vi "期末專題_R09522534_楊日昌.vi"() -> ()   [LabVIEW 2014]
uses:
  <vilib>/Utility/miscctls.llb/LVPositionTypeDef.ctl
  <vilib>/Utility/inputDevices.llb/keyboardAcquire.vi
panel:
  out "test":dbl
  out "撞擊次數2":dbl
  out "撞擊次數1":dbl
  out "操作模式":string
  out "操作模式":string
  in  "stop":bool
  out "Ball 3":bool
  out "Ball 2":bool
  out "最佳成績":dbl
  out "judge2":dbl
  out "分數":dbl
  out "選擇的模式2":dbl
  out "judge1":dbl
  out "選擇的模式1":dbl
  in  "Boolean":bool=TRUE
  out "bowling5":bool=TRUE
  out "bowling4":bool=TRUE
  out "時間":dbl
  out "Ball":bool=TRUE
  out "碰撞次數(以內)":dbl
  out "bowling3":bool=TRUE
  out "bowling2":bool=TRUE
  in  "START":bool
  out "bowling1":bool=TRUE
  in  "Dial":dbl(knob)
  # "保齡撞撞樂"
  # "加分任務"
  # "操作及模式"
  # "出球"
  # "移動"
  # "角度"
  # "操作模式"
  # ":"
  # "剩餘球數"
types:
  T1 = typedef "LVPositionTypeDef.ctl" = cluster{"Left":i32, "Top":i32}
  T2 = enum16{"0", "1", "2", "3", "4", "5", "6", "7", "8", "9", "A", "B", "C", "D", "E", "F", "G", "H", "I", "J", "K", "L", "M", "N", "O", "P", "Q", "R", "S", "T", "U", "V", "W", "X", "Y", "Z", "F1", "F2", "F3", "F4", "F5", "F6", "F7", "F8", "F9", "F10", "F11", "F12", "F13", "F14", "F15", "ADD", "BACK", "BACKSLASH", "CAPITAL", "COMMA", "DECIMAL", "DELETE", "DIVIDE", "DOWN", "END", "EQUALS", "ESCAPE", "GRAVE (`)", "HOME", "INSERT", "LBRACKET", "LCONTROL", "LEFT", "L ALT", "LSHIFT", "LWIN", "MINUS", "MULTIPLY", "NEXT", "NUMLOCK", "NUMPAD_0", "NUMPAD_1", "NUMPAD_2", "NUMPAD_3", "NUMPAD_4", "NUMPAD_5", "NUMPAD_6", "NUMPAD_7", "NUMPAD_8", "NUMPAD_9", "PAUSE", "PERIOD", "PRIOR (PG UP)", "RBRACKET", "RCONTROL", "RETURN", "RIGHT", "R ALT", "RSHIFT", "RWIN", "SCROLL", "SEMICOLON", "SLASH", "SPACE", "SUBTRACT", "TAB", "UP", "ENTER (num pad)", "' (quote)"}[]
  T3 = enum16{"0", "1", "2", "3", "4", "5", "6", "7", "8", "9", "A", "B", "C", "D", "E", "F", "G", "H", "I", "J", "K", "L", "M", "N", "O", "P", "Q", "R", "S", "T", "U", "V", "W", "X", "Y", "Z", "F1", "F2", "F3", "F4", "F5", "F6", "F7", "F8", "F9", "F10", "F11", "F12", "F13", "F14", "F15", "ADD", "BACK", "BACKSLASH", "CAPITAL", "COMMA", "DECIMAL", "DELETE", "DIVIDE", "DOWN", "END", "EQUALS", "ESCAPE", "GRAVE (`)", "HOME", "INSERT", "LBRACKET", "LCONTROL", "LEFT", "L ALT", "LSHIFT", "LWIN", "MINUS", "MULTIPLY", "NEXT", "NUMLOCK", "NUMPAD_0", "NUMPAD_1", "NUMPAD_2", "NUMPAD_3", "NUMPAD_4", "NUMPAD_5", "NUMPAD_6", "NUMPAD_7", "NUMPAD_8", "NUMPAD_9", "PAUSE", "PERIOD", "PRIOR (PG UP)", "RBRACKET", "RCONTROL", "RETURN", "RIGHT", "R ALT", "RSHIFT", "RWIN", "SCROLL", "SEMICOLON", "SLASH", "SPACE", "SUBTRACT", "TAB", "UP", "ENTER (num pad)", "' (quote)"}
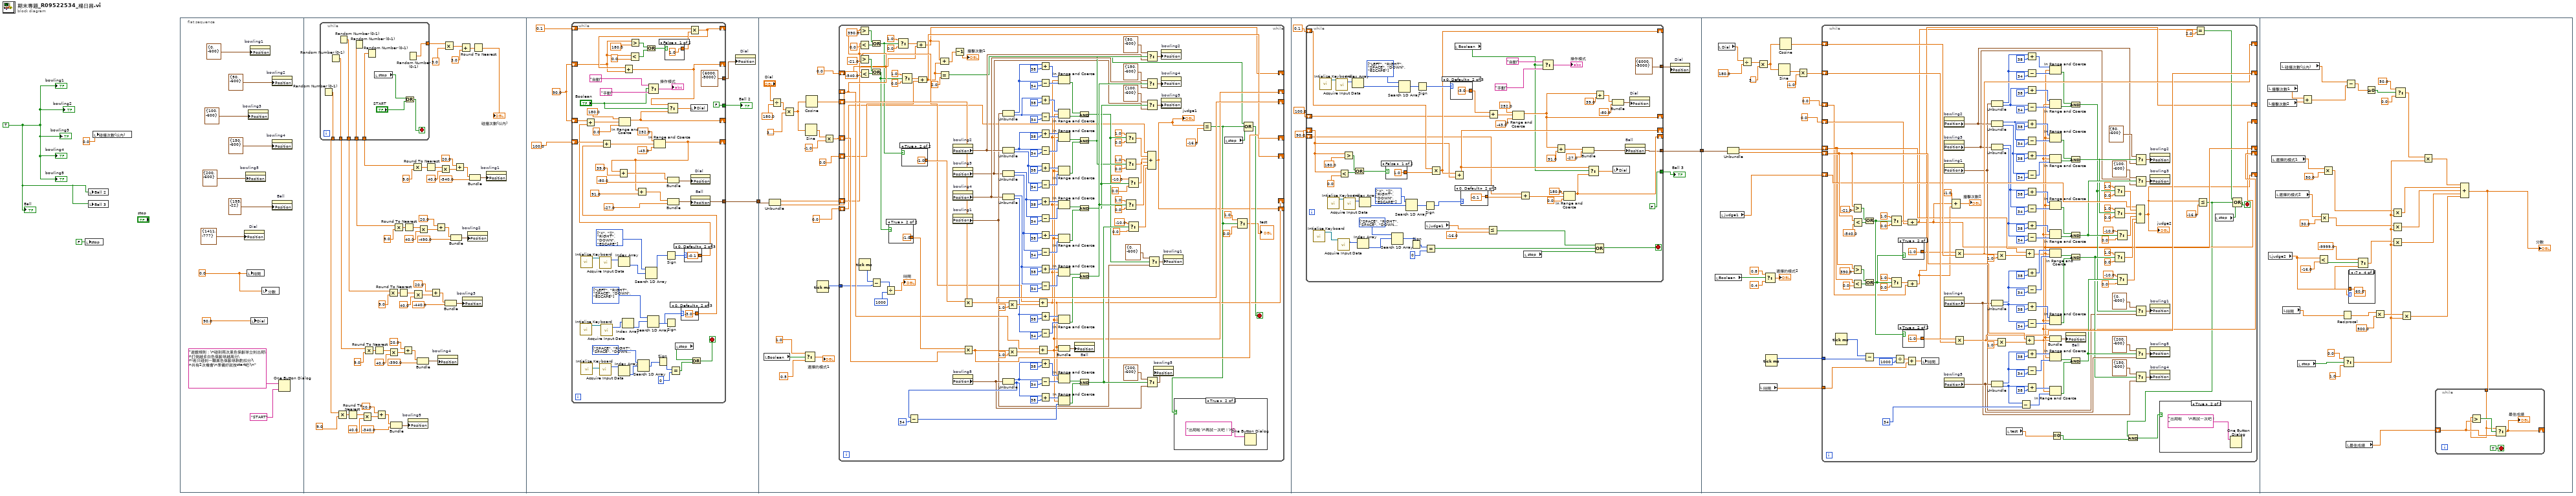
[diagram p0: block diagram]
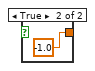
[diagram p2: hidden frame]
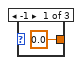
[diagram p3: hidden frame]
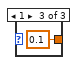
[diagram p4: hidden frame]
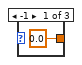
[diagram p5: hidden frame]
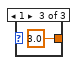
[diagram p6: hidden frame]
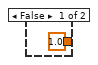
[diagram p8: hidden frame]
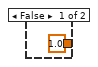
[diagram p9: hidden frame]
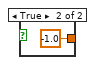
[diagram p10: hidden frame]
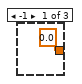
[diagram p11: hidden frame]
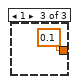
[diagram p12: hidden frame]
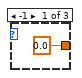
[diagram p13: hidden frame]
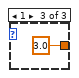
[diagram p14: hidden frame]
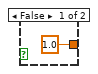
[diagram p16: hidden frame]
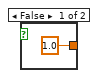
[diagram p17: hidden frame]
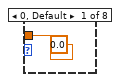
[diagram p18: hidden frame]
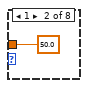
[diagram p19: hidden frame]
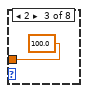
[diagram p20: hidden frame]
diagram:
  w1 = TRUE
  n1 = local write "stop"(FALSE ("stop")) -> ()
  n2 = local write "Ball 2"(w1) -> ()
  n3 = local write "Ball 3"(w1) -> ()
  n4 = local write "碰撞次數(以內)"(0.0 ("Bouncing")) -> ()
  n5 = flat-sequence {
    tunnel: [w86] -> w5
    tunnel: w5 -> [w174]
    tunnel: [w329] -> w4
    tunnel: w4 -> [w414]
    frame #0 {
      w8 = 0.0 ("Time")
      n6 = property on="Dial" class="Knob (strict)"("Position"=T1 {"Left"=1411, "Top"=-777}) -> ()  [unwired: 2 in, 2 out]
      n7 = property on="bowling5" class="Bool (strict)"("Position"=T1 {"Left"=200, "Top"=-600}) -> ()  [unwired: 2 in, 2 out]
      n8 = local write "時間"(w8) -> ()
      n9 = property on="bowling3" class="Bool (strict)"("Position"=T1 {"Left"=100, "Top"=-600}) -> ()  [unwired: 2 in, 2 out]
      n10 = property on="bowling1" class="Bool (strict)"("Position"=T1 {"Left"=0, "Top"=-600}) -> ()  [unwired: 2 in, 2 out]
      n11 = local write "Dial"(90.0 ("Gauge")) -> ()
      n12 = local write "分數"(w8) -> ()
      n13 = property on="bowling2" class="Bool (strict)"("Position"=T1 {"Left"=50, "Top"=-600}) -> ()  [unwired: 2 in, 2 out]
      n14 = property on="bowling4" class="Bool (strict)"("Position"=T1 {"Left"=150, "Top"=-600}) -> ()  [unwired: 2 in, 2 out]
      n15 = property on="Ball" class="Bool (strict)"("Position"=T1 {"Left"=195, "Top"=-22}) -> ()  [unwired: 2 in, 2 out]
      n16 = One Button Dialog(message="遊戲規則：\n碰到兩次黑色保齡球立刻出局\n打倒越多白色保齡球越高分\n(若只碰到一顆黑色保齡球斟酌扣分)\n共有2次機會\n準備好就按start吧!\n" ("String"), button name ("OK")="START") -> ()  [unwired: 1 out]
    }
    frame #1 {
      n17 = while {
        tunnel: [w81] -> w49
        tunnel: [w80] -> w51
        tunnel: [w79] -> w50
        tunnel: [w78] -> w41
        tunnel: [w77] -> w18
        tunnel: [w76] -> w17
        stop <- w73 stop-if-true
        n18 = Random Number (0-1)() -> (number: 0 to 1=w76:dbl)
        n19 = Random Number (0-1)() -> (number: 0 to 1=w77:dbl)
        n20 = Random Number (0-1)() -> (number: 0 to 1=w80:dbl)
        n21 = Random Number (0-1)() -> (number: 0 to 1=w79:dbl)
        n22 = Random Number (0-1)() -> (number: 0 to 1=w81:dbl)
        n23 = local read "stop"() -> (w75:bool)
        n24 = Or(x=w75, y="START") -> (x .or. y?=w73:bool)
        n25 = Random Number (0-1)() -> (number: 0 to 1=w78:dbl)
      }
      n26 = Multiply(x=w17, y=9.0) -> (x*y=w22:dbl)
      n27 = Round To Nearest(number=w22) -> (nearest integer value=w21:dbl)
      n28 = Multiply(x=w21, y=40.0) -> (x*y=w25:dbl)
      n29 = Multiply(x=w18, y=9.0) -> (x*y=w35:dbl)
      n30 = Round To Nearest(number=w35) -> (nearest integer value=w36:dbl)
      n31 = Add(x=20.0, y=w25) -> (x+y=w26:dbl)
      n32 = Multiply(x=w51, y=9.0) -> (x*y=w44:dbl)
      n33 = Multiply(x=w36, y=40.0) -> (x*y=w32:dbl)
      n34 = Bundle(w26, "x"=-340.0) -> (w19:cluster{dbl, "x":dbl})  [unwired: 1 in]
      n35 = Multiply(x=w50, y=9.0) -> (x*y=w46:dbl)
      n36 = Round To Nearest(number=w44) -> (nearest integer value=w43:dbl)
      n37 = Add(x=20.0, y=w32) -> (x+y=w31:dbl)
      n38 = Round To Nearest(number=w46) -> (nearest integer value=w45:dbl)
      n39 = property on="bowling5" class="Bool (strict)"("Position"=w19) -> ()  [unwired: 2 in, 2 out]
      n40 = Multiply(x=w49, y=9.0) -> (x*y=w48:dbl)
      n41 = Multiply(x=w43, y=40.0) -> (x*y=w58:dbl)
      n42 = Bundle(w31, "x"=-390.0) -> (w20:cluster{dbl, "x":dbl})  [unwired: 1 in]
      n43 = Multiply(x=w45, y=40.0) -> (x*y=w65:dbl)
      n44 = Round To Nearest(number=w48) -> (nearest integer value=w47:dbl)
      n45 = Add(x=20.0, y=w58) -> (x+y=w59:dbl)
      n46 = Add(x=20.0, y=w65) -> (x+y=w64:dbl)
      n47 = property on="bowling4" class="Bool (strict)"("Position"=w20) -> ()  [unwired: 2 in, 2 out]
      n48 = Multiply(x=w47, y=40.0) -> (x*y=w68:dbl)
      n49 = Multiply(x=w41, y=3.0) -> (x*y=w38:dbl)
      n50 = Bundle(w59, "x"=-440.0) -> (w55:cluster{dbl, "x":dbl})  [unwired: 1 in]
      n51 = Bundle(w64, "x"=-490.0) -> (w56:cluster{dbl, "x":dbl})  [unwired: 1 in]
      n52 = Add(x=20.0, y=w68) -> (x+y=w70:dbl)
      n53 = Add(x=w38, y=3.0) -> (x+y=w39:dbl)
      n54 = property on="bowling3" class="Bool (strict)"("Position"=w55) -> ()  [unwired: 2 in, 2 out]
      n55 = property on="bowling2" class="Bool (strict)"("Position"=w56) -> ()  [unwired: 2 in, 2 out]
      n56 = Bundle(w70, "x"=-540.0) -> (w69:cluster{dbl, "x":dbl})  [unwired: 1 in]
      n57 = Round To Nearest(number=w39) -> (nearest integer value=→"碰撞次數(以內)":dbl)
      n58 = property on="bowling1" class="Bool (strict)"("Position"=w69) -> ()  [unwired: 2 in, 2 out]
    }
    frame #2 {
      w83 = 90.0
      n59 = while {
        shift-right: [w93] -> _
        shift-left: 100.0 -> [w104]
        tunnel: [w116] -> w86
        shift-right: [w114] -> _
        shift-left: w83 -> [w103]
        tunnel: [T1 {"Left"=6000, "Top"=-5000} ("Position")] -> w82
        shift-right: [w89] -> _
        shift-left: w83 -> [w100]
        shift-right: [w101] -> _
        shift-left: 0.1 -> [w107]
        tunnel: [FALSE ("Ball 2")] -> w84
        stop <- w95 stop-if-true
        w121 = T2 [enum."SPACE", enum."RIGHT", enum."SPACE", enum."DOWN", enum."ESCAPE"] items=["0", "1", "2", "3", "4", "5", "6", "7", "8", "9", "A", "B", "C", "D", "E", "F", "G", "H", "I", "J", "K", "L", "M", "N", "O", "P", "Q", "R", "S", "T", "U", "V", "W", "X", "Y", "Z", "F1", "F2", "F3", "F4", "F5", "F6", "F7", "F8", "F9", "F10", "F11", "F12", "F13", "F14", "F15", "ADD", "BACK", "BACKSLASH", "CAPITAL", "COMMA", "DECIMAL", "DELETE", "DIVIDE", "DOWN", "END", "EQUALS", "ESCAPE", "GRAVE (`)", "HOME", "INSERT", "LBRACKET", "LCONTROL", "LEFT", "L ALT", "LSHIFT", "LWIN", "MINUS", "MULTIPLY", "NEXT", "NUMLOCK", "NUMPAD_0", "NUMPAD_1", "NUMPAD_2", "NUMPAD_3", "NUMPAD_4", "NUMPAD_5", "NUMPAD_6", "NUMPAD_7", "NUMPAD_8", "NUMPAD_9", "PAUSE", "PERIOD", "PRIOR (PG UP)", "RBRACKET", "RCONTROL", "RETURN", "RIGHT", "R ALT", "RSHIFT", "RWIN", "SCROLL", "SEMICOLON", "SLASH", "SPACE", "SUBTRACT", "TAB", "UP", "ENTER (num pad)", "' (quote)"] ("keys pressed 2")
        w132 = T2 [enum."X", enum."Z", enum."RIGHT", enum."DOWN", enum."ESCAPE"] items=["0", "1", "2", "3", "4", "5", "6", "7", "8", "9", "A", "B", "C", "D", "E", "F", "G", "H", "I", "J", "K", "L", "M", "N", "O", "P", "Q", "R", "S", "T", "U", "V", "W", "X", "Y", "Z", "F1", "F2", "F3", "F4", "F5", "F6", "F7", "F8", "F9", "F10", "F11", "F12", "F13", "F14", "F15", "ADD", "BACK", "BACKSLASH", "CAPITAL", "COMMA", "DECIMAL", "DELETE", "DIVIDE", "DOWN", "END", "EQUALS", "ESCAPE", "GRAVE (`)", "HOME", "INSERT", "LBRACKET", "LCONTROL", "LEFT", "L ALT", "LSHIFT", "LWIN", "MINUS", "MULTIPLY", "NEXT", "NUMLOCK", "NUMPAD_0", "NUMPAD_1", "NUMPAD_2", "NUMPAD_3", "NUMPAD_4", "NUMPAD_5", "NUMPAD_6", "NUMPAD_7", "NUMPAD_8", "NUMPAD_9", "PAUSE", "PERIOD", "PRIOR (PG UP)", "RBRACKET", "RCONTROL", "RETURN", "RIGHT", "R ALT", "RSHIFT", "RWIN", "SCROLL", "SEMICOLON", "SLASH", "SPACE", "SUBTRACT", "TAB", "UP", "ENTER (num pad)", "' (quote)"] ("keys pressed 2")
        w143 = T2 [enum."LEFT", enum."RIGHT", enum."SPACE", enum."DOWN", enum."ESCAPE"] items=["0", "1", "2", "3", "4", "5", "6", "7", "8", "9", "A", "B", "C", "D", "E", "F", "G", "H", "I", "J", "K", "L", "M", "N", "O", "P", "Q", "R", "S", "T", "U", "V", "W", "X", "Y", "Z", "F1", "F2", "F3", "F4", "F5", "F6", "F7", "F8", "F9", "F10", "F11", "F12", "F13", "F14", "F15", "ADD", "BACK", "BACKSLASH", "CAPITAL", "COMMA", "DECIMAL", "DELETE", "DIVIDE", "DOWN", "END", "EQUALS", "ESCAPE", "GRAVE (`)", "HOME", "INSERT", "LBRACKET", "LCONTROL", "LEFT", "L ALT", "LSHIFT", "LWIN", "MINUS", "MULTIPLY", "NEXT", "NUMLOCK", "NUMPAD_0", "NUMPAD_1", "NUMPAD_2", "NUMPAD_3", "NUMPAD_4", "NUMPAD_5", "NUMPAD_6", "NUMPAD_7", "NUMPAD_8", "NUMPAD_9", "PAUSE", "PERIOD", "PRIOR (PG UP)", "RBRACKET", "RCONTROL", "RETURN", "RIGHT", "R ALT", "RSHIFT", "RWIN", "SCROLL", "SEMICOLON", "SLASH", "SPACE", "SUBTRACT", "TAB", "UP", "ENTER (num pad)", "' (quote)"] ("keys pressed 2")
        n60 = call <vilib>:"Intialize Keyboard.vi"() -> ("device ID"=w144:refnum<k1>)  [unwired: 10 in, 1 out]
        n61 = call <vilib>:"Intialize Keyboard.vi"() -> ("device ID"=w125:refnum<k1>)  [unwired: 10 in, 1 out]
        n62 = call <vilib>:"Intialize Keyboard.vi"() -> ("device ID"=w120:refnum<k1>)  [unwired: 10 in, 1 out]
        n63 = call-poly <vilib>:"Acquire Input Data.vi"("device ID"=w120) -> ("keys pressed"=w122:T2)  [unwired: 16 in, 2 out]
        n64 = call-poly <vilib>:"Acquire Input Data.vi"("device ID"=w125) -> ("keys pressed"=w126:T2)  [unwired: 16 in, 2 out]
        n65 = call-poly <vilib>:"Acquire Input Data.vi"("device ID"=w144) -> ("keys pressed"=w142:T2)  [unwired: 16 in, 2 out]
        n66 = Index Array(array=w122) -> (element=w123:T3)  [unwired: 1 in]
        n67 = Index Array(array=w126) -> (element=w124:T3)  [unwired: 1 in]
        n68 = Index Array(array=w142) -> (element=w133:T3)  [unwired: 1 in]
        n69 = Less?(x=w100, y=0.0) -> (x < y?=w111:bool)
        n70 = Greater?(x=w100, y=180.0) -> (0:w110:bool)
        n71 = Search 1D Array(1D array=w121, element=w123) -> (index of element=w119:i32)  [unwired: 1 in]
        n72 = Search 1D Array(1D array=w132, element=w124) -> (index of element=w131:i32)  [unwired: 1 in]
        n73 = Or(x=w110, y=w111) -> (x .or. y?=w108:bool)
        n74 = Search 1D Array(1D array=w143, element=w133) -> (index of element=w145:i32)  [unwired: 1 in]
        n75 = Select(t="自動", s="Boolean", f="手動") -> (s? t:f=→"操作模式":string)
        n76 = Sign(1:w119) -> (0:w118:i32)
        n77 = case shown="False" w108 {
          tunnel: [1.0 -1.0] -> w113
          frame False {
          }
          frame True {
          }
        }
        n78 = Sign(1:w131) -> (0:w127:i32)
        n79 = Sign(1:w145) -> (0:w146:i32)
        n80 = Equal?(x=w118, y=0) -> (x = y?=w96:bool)
        n81 = local read "stop"() -> (w97:bool)
        n82 = case shown="0, Default" w146 {
          tunnel: [0.0 -3.0 3.0] -> w94
          frame -1 {
          }
          frame 0, Default {
          }
          frame 1 {
          }
        }
        n83 = Add(x=w104, y=w94) -> (x+y=w138:dbl)
        n84 = In Range and Coerce(upper limit=252.0, x=w138, lower limit=-43.0) -> (coerced(x)=w93:dbl)  [unwired: 1 out]
        n85 = Add(x=w93, y=39.0) -> (x+y=w105:dbl)
        n86 = Add(x=w93, y=91.0) -> (x+y=w136:dbl)
        n87 = Bundle(w105, -80.0) -> (w137:cluster{dbl, dbl})  [unwired: 1 in]
        n88 = Bundle(w136, -27.0) -> (w116:cluster{dbl, dbl})  [unwired: 1 in]
        n89 = case shown="0, Default" w127 {
          tunnel: [0.0 -0.1 0.1] -> w102
          frame -1 {
          }
          frame 0, Default {
          }
          frame 1 {
          }
        }
        n90 = Add(x=w103, y=w102) -> (x+y=w130:dbl)
        n91 = In Range and Coerce(upper limit=180.0, x=w130, lower limit=0.0) -> (coerced(x)=w114:dbl)  [unwired: 1 out]
        n92 = Multiply(x=w107, y=w113) -> (x*y=w101:dbl)
        n93 = Add(x=w101, y=w100) -> (x+y=w89:dbl)
        n94 = Select(t=w89, s="Boolean", f=w114) -> (s? t:f=w99:dbl)
        n95 = local write "Dial"(w99) -> ()
        n96 = property on="Dial" class="Knob (strict)"("Position"=w137) -> ()  [unwired: 2 in, 2 out]
        n97 = property on="Ball" class="Bool (strict)"("Position"=w116) -> ()  [unwired: 2 in, 2 out]
        n98 = Or(x=w97, y=w96) -> (x .or. y?=w95:bool)
      }
      "Ball 2" <- w84
      n99 = property on="Dial" class="Knob (strict)"("Position"=w82) -> ()  [unwired: 2 in, 2 out]
    }
    frame #3 {
      n100 = local read "Boolean"() -> (w158:bool)
      n101 = Unbundle(w174) -> (w159:dbl, w173:dbl)
      n102 = Divide(x="Dial", y=180.0) -> (x/y=w170:dbl)
      n103 = Multiply(x=w170, y=3.141592653589793) -> (x*y=w168:dbl)
      n104 = Select(t=1.0, s=w158, f=0.5) -> (s? t:f=→"選擇的模式1":dbl)
      n105 = Sine(x=w168) -> (sin(x)=w166:dbl)
      n106 = Cosine(x=w168) -> (cos(x)=w160:dbl)
      n107 = Tick Count (ms)() -> (millisecond timer value=w163:u32)
      n108 = Multiply(x=w166, y=-1.0) -> (x*y=w165:dbl)
      n109 = while {
        shift-right: [w198] -> _
        shift-left: w159 -> [w194]
        shift-right: [w305] -> _
        shift-left: w160 -> [w319]
        shift-right: [w199] -> _
        shift-left: w173 -> [w311]
        shift-right: [w307] -> _
        shift-left: w165 -> [w312]
        shift-right: [w184] -> _
        shift-left: 0.0 ("y") -> [w185]
        tunnel: w163 -> [w287]
        shift-right: [w182] -> _
        shift-left: 0.0 ("f") -> [w192]
        shift-right: [w181] -> _
        shift-left: 0.0 ("f") -> [w190]
        stop <- w186 stop-if-true
        n110 = Greater?(x=w194, y=390.0) -> (0:w321:bool)
        n111 = Less?(x=w194, y=0.0) -> (x < y?=w320:bool)
        n112 = Greater?(x=w311, y=-21.0) -> (0:w315:bool)
        n113 = Tick Count (ms)() -> (millisecond timer value=w288:u32)
        n114 = Less?(x=w311, y=-540.0) -> (x < y?=w314:bool)
        n115 = Or(x=w321, y=w320) -> (x .or. y?=w196:bool)
        n116 = Or(x=w315, y=w314) -> (x .or. y?=w259:bool)
        n117 = Subtract(x=w288, y=w287) -> (x-y=w286:u32)
        n118 = Divide(x=w286, y=u32 1000) -> (x/y=→"時間":dbl)
        n119 = case shown="True" w259 {
          tunnel: [1.0 -1.0] -> w313
          frame False {
          }
          frame True {
          }
        }
        n120 = Select(t=1.0, s=w196, f=0.0) -> (s? t:f=w191:dbl)
        n121 = Select(t=1.0, s=w259, f=0.0) -> (s? t:f=w193:dbl)
        n122 = case shown="True" w196 {
          tunnel: [1.0 -1.0] -> w195
          frame False {
          }
          frame True {
          }
        }
        n123 = Compound Arithmetic op=ADD(w191, w190) -> (w181:dbl)
        n124 = Compound Arithmetic op=ADD(w193, w192) -> (w182:dbl)
        n125 = Equal?(x=w182, y=2.0) -> (x = y?=w187:bool)
        n126 = Compound Arithmetic op=ADD(w181, w182) -> (w180:dbl)
        n127 = property on="bowling2" class="Bool (strict)"() -> ("Position"=w214:T1)  [unwired: 2 in, 2 out]
        n128 = property on="bowling3" class="Bool (strict)"() -> ("Position"=w197:T1)  [unwired: 2 in, 2 out]
        n129 = property on="bowling4" class="Bool (strict)"() -> ("Position"=w241:T1)  [unwired: 2 in, 2 out]
        n130 = property on="bowling1" class="Bool (strict)"() -> ("Position"=w200:T1)  [unwired: 2 in, 2 out]
        n131 = property on="bowling5" class="Bool (strict)"() -> ("Position"=w269:T1)  [unwired: 2 in, 2 out]
        n132 = Decrement(x=w180) -> (x-1=→"撞擊次數1":dbl)
        n133 = Multiply(x=w195, y=w319) -> (x*y=w305:dbl)
        n134 = Multiply(x=w313, y=w312) -> (x*y=w307:dbl)
        n135 = Unbundle(w200) -> ("Left"=w207:i32, "Top"=w212:i32)
        n136 = Unbundle(w214) -> ("Left"=w221:i32, "Top"=w226:i32)
        n137 = Unbundle(w197) -> ("Left"=w234:i32, "Top"=w239:i32)
        n138 = Unbundle(w241) -> ("Left"=w243:i32, "Top"=w242:i32)
        n139 = Unbundle(w269) -> ("Left"=w276:i32, "Top"=w281:i32)
        n140 = Subtract(x=w281, y=34) -> (x-y=w277:i32)
        n141 = Multiply(x=w305, y=1.0) -> (x*y=w306:dbl)
        n142 = Multiply(x=w307, y=1.0) -> (x*y=w308:dbl)
        n143 = Add(x=w194, y=w306) -> (x+y=w198:dbl)
        n144 = Add(x=w311, y=w308) -> (x+y=w199:dbl)
        n145 = Add(x=w207, y=38) -> (x+y=w211:i32)
        n146 = Subtract(x=w207, y=34) -> (x-y=w206:i32)
        n147 = Add(x=w212, y=38) -> (x+y=w210:i32)
        n148 = Subtract(x=w212, y=34) -> (x-y=w208:i32)
        n149 = Add(x=w221, y=38) -> (x+y=w225:i32)
        n150 = Subtract(x=w221, y=34) -> (x-y=w220:i32)
        n151 = Add(x=w226, y=38) -> (x+y=w224:i32)
        n152 = Subtract(x=w226, y=34) -> (x-y=w222:i32)
        n153 = Add(x=w234, y=38) -> (x+y=w238:i32)
        n154 = Subtract(x=w234, y=34) -> (x-y=w233:i32)
        n155 = Add(x=w239, y=38) -> (x+y=w237:i32)
        n156 = Subtract(x=w239, y=34) -> (x-y=w235:i32)
        n157 = Add(x=w243, y=38) -> (x+y=w253:i32)
        n158 = Subtract(x=w243, y=34) -> (x-y=w249:i32)
        n159 = Add(x=w242, y=38) -> (x+y=w252:i32)
        n160 = Subtract(x=w242, y=34) -> (x-y=w250:i32)
        n161 = Add(x=w276, y=38) -> (x+y=w280:i32)
        n162 = Subtract(x=w276, y=34) -> (x-y=w275:i32)
        n163 = Add(x=w281, y=38) -> (x+y=w279:i32)
        n164 = In Range and Coerce(upper limit=w211, x=w198, lower limit=w206) -> (In Range?=w202:bool)  [unwired: 1 out]
        n165 = In Range and Coerce(upper limit=w210, x=w199, lower limit=w208) -> (In Range?=w203:bool)  [unwired: 1 out]
        n166 = In Range and Coerce(upper limit=w225, x=w198, lower limit=w220) -> (In Range?=w216:bool)  [unwired: 1 out]
        n167 = In Range and Coerce(upper limit=w224, x=w199, lower limit=w222) -> (In Range?=w217:bool)  [unwired: 1 out]
        n168 = In Range and Coerce(upper limit=w238, x=w198, lower limit=w233) -> (In Range?=w229:bool)  [unwired: 1 out]
        n169 = In Range and Coerce(upper limit=w237, x=w199, lower limit=w235) -> (In Range?=w230:bool)  [unwired: 1 out]
        n170 = In Range and Coerce(upper limit=w253, x=w198, lower limit=w249) -> (In Range?=w245:bool)  [unwired: 1 out]
        n171 = In Range and Coerce(upper limit=w252, x=w199, lower limit=w250) -> (In Range?=w246:bool)  [unwired: 1 out]
        n172 = Bundle(w198, w199) -> (w304:cluster{dbl, dbl})  [unwired: 1 in]
        n173 = In Range and Coerce(upper limit=w280, x=w198, lower limit=w275) -> (In Range?=w271:bool)  [unwired: 1 out]
        n174 = In Range and Coerce(upper limit=w279, x=w199, lower limit=w277) -> (In Range?=w272:bool)  [unwired: 1 out]
        n175 = property on="Ball" class="Bool (strict)"("Position"=w304) -> ()  [unwired: 2 in, 2 out]
        n176 = And(x=w202, y=w203) -> (x .and. y?=w201:bool)
        n177 = And(x=w216, y=w217) -> (x .and. y?=w215:bool)
        n178 = And(x=w229, y=w230) -> (x .and. y?=w228:bool)
        n179 = And(x=w245, y=w246) -> (x .and. y?=w244:bool)
        n180 = And(x=w271, y=w272) -> (x .and. y?=w264:bool)
        n181 = Select(t=1.0, s=w201, f=0.0) -> (s? t:f=w291:dbl)
        n182 = Select(t=1.0, s=w215, f=0.0) -> (s? t:f=w290:dbl)
        n183 = Select(t=1.0, s=w244, f=0.0) -> (s? t:f=w263:dbl)
        n184 = Select(t=-10.0, s=w228, f=0.0) -> (s? t:f=w289:dbl)
        n185 = Select(t=-10.0, s=w264, f=0.0) -> (s? t:f=w262:dbl)
        n186 = Select(t=T1 {"Left"=50, "Top"=-600}, s=w215, f=w214) -> (s? t:f=w299:T1)
        n187 = Select(t=T1 {"Left"=150, "Top"=-600}, s=w244, f=w241) -> (s? t:f=w261:T1)
        n188 = Select(t=T1 {"Left"=100, "Top"=-600}, s=w228, f=w197) -> (s? t:f=w298:T1)
        n189 = Select(t=T1 {"Left"=200, "Top"=-600}, s=w264, f=w269) -> (s? t:f=w260:T1)
        n190 = Compound Arithmetic op=ADD(w185, w291, w290, w289, w263, w262) -> (w184:dbl)
        "judge1" <- w184
        n191 = Select(t=T1 {"Left"=0, "Top"=-600}, s=w201, f=w200) -> (s? t:f=w302:T1)
        n192 = property on="bowling5" class="Bool (strict)"("Position"=w260) -> ()  [unwired: 2 in, 2 out]
        n193 = property on="bowling2" class="Bool (strict)"("Position"=w299) -> ()  [unwired: 2 in, 2 out]
        n194 = property on="bowling4" class="Bool (strict)"("Position"=w261) -> ()  [unwired: 2 in, 2 out]
        n195 = property on="bowling3" class="Bool (strict)"("Position"=w298) -> ()  [unwired: 2 in, 2 out]
        n196 = property on="bowling1" class="Bool (strict)"("Position"=w302) -> ()  [unwired: 2 in, 2 out]
        n197 = Less Or Equal?(x=w184, y=-16.0) -> (x <= y?=w177:bool)
        n198 = case shown="True" w177 {
          frame False {
          }
          frame True {
            n199 = One Button Dialog(message="出局啦 \n再試一次吧！\n") -> ()  [unwired: 1 in, 1 out]
          }
        }
        n200 = local read "stop"() -> (w188:bool)
        n201 = Select(t=1.0, s=w177, f=0.0) -> (s? t:f=→"test":dbl)
        n202 = Compound Arithmetic op=OR(w187, w177, w188) -> (w186:bool)
      }
    }
    frame #4 {
      w331 = 90.0
      n203 = while {
        shift-right: [w352] -> _
        shift-left: 100.0 -> [w337]
        tunnel: [w335] -> w329
        shift-right: [w363] -> _
        shift-left: w331 -> [w338]
        tunnel: [T1 {"Left"=6000, "Top"=-5000} ("Position")] -> w332
        shift-right: [w364] -> _
        shift-left: w331 -> [w349]
        shift-right: [w350] -> _
        shift-left: 0.1 -> [w356]
        tunnel: [FALSE ("Ball 3")] -> w328
        stop <- w345 stop-if-true
        w370 = T2 [enum."SPACE", enum."RIGHT", enum."SPACE", enum."DOWN", enum."ESCAPE"] items=["0", "1", "2", "3", "4", "5", "6", "7", "8", "9", "A", "B", "C", "D", "E", "F", "G", "H", "I", "J", "K", "L", "M", "N", "O", "P", "Q", "R", "S", "T", "U", "V", "W", "X", "Y", "Z", "F1", "F2", "F3", "F4", "F5", "F6", "F7", "F8", "F9", "F10", "F11", "F12", "F13", "F14", "F15", "ADD", "BACK", "BACKSLASH", "CAPITAL", "COMMA", "DECIMAL", "DELETE", "DIVIDE", "DOWN", "END", "EQUALS", "ESCAPE", "GRAVE (`)", "HOME", "INSERT", "LBRACKET", "LCONTROL", "LEFT", "L ALT", "LSHIFT", "LWIN", "MINUS", "MULTIPLY", "NEXT", "NUMLOCK", "NUMPAD_0", "NUMPAD_1", "NUMPAD_2", "NUMPAD_3", "NUMPAD_4", "NUMPAD_5", "NUMPAD_6", "NUMPAD_7", "NUMPAD_8", "NUMPAD_9", "PAUSE", "PERIOD", "PRIOR (PG UP)", "RBRACKET", "RCONTROL", "RETURN", "RIGHT", "R ALT", "RSHIFT", "RWIN", "SCROLL", "SEMICOLON", "SLASH", "SPACE", "SUBTRACT", "TAB", "UP", "ENTER (num pad)", "' (quote)"] ("keys pressed 2")
        w381 = T2 [enum."X", enum."Z", enum."RIGHT", enum."DOWN", enum."ESCAPE"] items=["0", "1", "2", "3", "4", "5", "6", "7", "8", "9", "A", "B", "C", "D", "E", "F", "G", "H", "I", "J", "K", "L", "M", "N", "O", "P", "Q", "R", "S", "T", "U", "V", "W", "X", "Y", "Z", "F1", "F2", "F3", "F4", "F5", "F6", "F7", "F8", "F9", "F10", "F11", "F12", "F13", "F14", "F15", "ADD", "BACK", "BACKSLASH", "CAPITAL", "COMMA", "DECIMAL", "DELETE", "DIVIDE", "DOWN", "END", "EQUALS", "ESCAPE", "GRAVE (`)", "HOME", "INSERT", "LBRACKET", "LCONTROL", "LEFT", "L ALT", "LSHIFT", "LWIN", "MINUS", "MULTIPLY", "NEXT", "NUMLOCK", "NUMPAD_0", "NUMPAD_1", "NUMPAD_2", "NUMPAD_3", "NUMPAD_4", "NUMPAD_5", "NUMPAD_6", "NUMPAD_7", "NUMPAD_8", "NUMPAD_9", "PAUSE", "PERIOD", "PRIOR (PG UP)", "RBRACKET", "RCONTROL", "RETURN", "RIGHT", "R ALT", "RSHIFT", "RWIN", "SCROLL", "SEMICOLON", "SLASH", "SPACE", "SUBTRACT", "TAB", "UP", "ENTER (num pad)", "' (quote)"] ("keys pressed 2")
        w392 = T2 [enum."LEFT", enum."RIGHT", enum."SPACE", enum."DOWN", enum."ESCAPE"] items=["0", "1", "2", "3", "4", "5", "6", "7", "8", "9", "A", "B", "C", "D", "E", "F", "G", "H", "I", "J", "K", "L", "M", "N", "O", "P", "Q", "R", "S", "T", "U", "V", "W", "X", "Y", "Z", "F1", "F2", "F3", "F4", "F5", "F6", "F7", "F8", "F9", "F10", "F11", "F12", "F13", "F14", "F15", "ADD", "BACK", "BACKSLASH", "CAPITAL", "COMMA", "DECIMAL", "DELETE", "DIVIDE", "DOWN", "END", "EQUALS", "ESCAPE", "GRAVE (`)", "HOME", "INSERT", "LBRACKET", "LCONTROL", "LEFT", "L ALT", "LSHIFT", "LWIN", "MINUS", "MULTIPLY", "NEXT", "NUMLOCK", "NUMPAD_0", "NUMPAD_1", "NUMPAD_2", "NUMPAD_3", "NUMPAD_4", "NUMPAD_5", "NUMPAD_6", "NUMPAD_7", "NUMPAD_8", "NUMPAD_9", "PAUSE", "PERIOD", "PRIOR (PG UP)", "RBRACKET", "RCONTROL", "RETURN", "RIGHT", "R ALT", "RSHIFT", "RWIN", "SCROLL", "SEMICOLON", "SLASH", "SPACE", "SUBTRACT", "TAB", "UP", "ENTER (num pad)", "' (quote)"] ("keys pressed 2")
        n204 = call <vilib>:"Intialize Keyboard.vi"() -> ("device ID"=w369:refnum<k1>)  [unwired: 10 in, 1 out]
        n205 = call <vilib>:"Intialize Keyboard.vi"() -> ("device ID"=w393:refnum<k1>)  [unwired: 10 in, 1 out]
        n206 = call <vilib>:"Intialize Keyboard.vi"() -> ("device ID"=w374:refnum<k1>)  [unwired: 10 in, 1 out]
        n207 = call-poly <vilib>:"Acquire Input Data.vi"("device ID"=w393) -> ("keys pressed"=w391:T2)  [unwired: 16 in, 2 out]
        n208 = call-poly <vilib>:"Acquire Input Data.vi"("device ID"=w369) -> ("keys pressed"=w371:T2)  [unwired: 16 in, 2 out]
        n209 = Less?(x=w349, y=0.0) -> (x < y?=w360:bool)
        n210 = Greater?(x=w349, y=180.0) -> (0:w359:bool)
        n211 = call-poly <vilib>:"Acquire Input Data.vi"("device ID"=w374) -> ("keys pressed"=w375:T2)  [unwired: 16 in, 2 out]
        n212 = Index Array(array=w391) -> (element=w382:T3)  [unwired: 1 in]
        n213 = Or(x=w359, y=w360) -> (x .or. y?=w357:bool)
        n214 = Index Array(array=w371) -> (element=w372:T3)  [unwired: 1 in]
        n215 = Index Array(array=w375) -> (element=w373:T3)  [unwired: 1 in]
        n216 = case shown="False" w357 {
          tunnel: [1.0 -1.0] -> w362
          frame False {
          }
          frame True {
          }
        }
        n217 = Search 1D Array(1D array=w370, element=w372) -> (index of element=w368:i32)  [unwired: 1 in]
        n218 = Search 1D Array(1D array=w392, element=w382) -> (index of element=w394:i32)  [unwired: 1 in]
        n219 = Search 1D Array(1D array=w381, element=w373) -> (index of element=w380:i32)  [unwired: 1 in]
        n220 = Sign(1:w368) -> (0:w367:i32)
        n221 = Sign(1:w394) -> (0:w395:i32)
        n222 = Sign(1:w380) -> (0:w376:i32)
        n223 = Equal?(x=w367, y=0) -> (x = y?=w344:bool)
        n224 = local read "judge1"() -> (w340:dbl)
        n225 = Multiply(x=w356, y=w362) -> (x*y=w350:dbl)
        n226 = case shown="0, Default" w395 {
          tunnel: [0.0 -3.0 3.0] -> w336
          frame -1 {
          }
          frame 0, Default {
          }
          frame 1 {
          }
        }
        n227 = Add(x=w350, y=w349) -> (x+y=w364:dbl)
        n228 = local read "Boolean"() -> (w348:bool)
        n229 = case shown="0, Default" w376 {
          tunnel: [0.0 -0.1 0.1] -> w351
          frame -1 {
          }
          frame 0, Default {
          }
          frame 1 {
          }
        }
        n230 = Less Or Equal?(x=w340, y=-16.0) -> (x <= y?=w339:bool)
        n231 = Add(x=w336, y=w337) -> (x+y=w387:dbl)
        n232 = In Range and Coerce(upper limit=252.0, x=w387, lower limit=-43.0) -> (coerced(x)=w352:dbl)  [unwired: 1 out]
        n233 = Add(x=w338, y=w351) -> (x+y=w379:dbl)
        n234 = local read "stop"() -> (w343:bool)
        n235 = Select(t="自動", s=w348, f="手動") -> (s? t:f=→"操作模式":string)
        n236 = Add(x=w352, y=91.0) -> (x+y=w385:dbl)
        n237 = In Range and Coerce(upper limit=180.0, x=w379, lower limit=0.0) -> (coerced(x)=w363:dbl)  [unwired: 1 out]
        n238 = Bundle(w385, -27.0) -> (w335:cluster{dbl, dbl})  [unwired: 1 in]
        n239 = Select(t=w364, s=w348, f=w363) -> (s? t:f=w347:dbl)
        n240 = Add(x=w352, y=39.0) -> (x+y=w353:dbl)
        n241 = Compound Arithmetic op=OR(w339, w344, w343) -> (w345:bool)
        n242 = Bundle(w353, -80.0) -> (w386:cluster{dbl, dbl})  [unwired: 1 in]
        n243 = local write "Dial"(w347) -> ()
        n244 = property on="Ball" class="Bool (strict)"("Position"=w335) -> ()  [unwired: 2 in, 2 out]
        n245 = property on="Dial" class="Knob (strict)"("Position"=w386) -> ()  [unwired: 2 in, 2 out]
      }
      "Ball 3" <- w328
      n246 = property on="Dial" class="Knob (strict)"("Position"=w332) -> ()  [unwired: 2 in, 2 out]
    }
    frame #5 {
      n247 = local read "Boolean"() -> (w409:bool)
      n248 = local read "Dial"() -> (w412:dbl)
      n249 = local read "judge1"() -> (w405:dbl)
      n250 = Unbundle(w414) -> (w424:dbl, w415:dbl)
      n251 = Divide(x=w412, y=180.0) -> (x/y=w417:dbl)
      n252 = Multiply(x=w417, y=3.141592653589793) -> (x*y=w419:dbl)
      n253 = local read "時間"() -> (w410:dbl)
      n254 = Select(t=0.8, s=w409, f=0.4) -> (s? t:f=→"選擇的模式2":dbl)
      n255 = Tick Count (ms)() -> (millisecond timer value=w413:u32)
      n256 = Sine(x=w419) -> (sin(x)=w421:dbl)
      n257 = Cosine(x=w419) -> (cos(x)=w423:dbl)
      n258 = Multiply(x=w421, y=-1.0) -> (x*y=w411:dbl)
      n259 = while {
        shift-right: [w450] -> _
        shift-left: w424 -> [w446]
        shift-right: [w557] -> _
        shift-left: w423 -> [w571]
        shift-right: [w451] -> _
        shift-left: w415 -> [w563]
        shift-right: [w559] -> _
        shift-left: w411 -> [w564]
        shift-right: [w429] -> _
        shift-left: w405 -> [w540]
        tunnel: w413 -> [w538]
        shift-right: [w432] -> _
        shift-left: 0.0 ("f") -> [w444]
        shift-right: [w433] -> _
        shift-left: 0.0 ("f") -> [w442]
        tunnel: w410 -> [w438]
        stop <- w437 stop-if-true
        n260 = Tick Count (ms)() -> (millisecond timer value=w539:u32)
        n261 = Greater?(x=w563, y=-21.0) -> (0:w567:bool)
        n262 = Greater?(x=w446, y=390.0) -> (0:w573:bool)
        n263 = Less?(x=w446, y=0.0) -> (x < y?=w572:bool)
        n264 = Less?(x=w563, y=-540.0) -> (x < y?=w566:bool)
        n265 = Or(x=w567, y=w566) -> (x .or. y?=w511:bool)
        n266 = Or(x=w573, y=w572) -> (x .or. y?=w448:bool)
        n267 = Subtract(x=w539, y=w538) -> (x-y=w537:u32)
        n268 = Select(t=1.0, s=w511, f=0.0) -> (s? t:f=w445:dbl)
        n269 = Select(t=1.0, s=w448, f=0.0) -> (s? t:f=w443:dbl)
        n270 = Divide(x=w537, y=u32 1000) -> (x/y=w440:dbl)
        n271 = case shown="True" w448 {
          tunnel: [1.0 -1.0] -> w447
          frame False {
          }
          frame True {
          }
        }
        n272 = case shown="True" w511 {
          tunnel: [1.0 -1.0] -> w565
          frame False {
          }
          frame True {
          }
        }
        n273 = Add(x=w440, y=w438) -> (x+y=w439:dbl)
        n274 = Compound Arithmetic op=ADD(w445, w444) -> (w432:dbl)
        n275 = Compound Arithmetic op=ADD(w443, w442) -> (w433:dbl)
        n276 = local write "時間"(w439) -> ()
        n277 = property on="bowling2" class="Bool (strict)"() -> ("Position"=w466:T1)  [unwired: 2 in, 2 out]
        n278 = property on="bowling3" class="Bool (strict)"() -> ("Position"=w449:T1)  [unwired: 2 in, 2 out]
        n279 = property on="bowling1" class="Bool (strict)"() -> ("Position"=w452:T1)  [unwired: 2 in, 2 out]
        n280 = property on="bowling4" class="Bool (strict)"() -> ("Position"=w493:T1)  [unwired: 2 in, 2 out]
        n281 = property on="bowling5" class="Bool (strict)"() -> ("Position"=w521:T1)  [unwired: 2 in, 2 out]
        n282 = Compound Arithmetic op=ADD(-1.0 ("value"), w432, w433) -> (→"撞擊次數2":dbl)
        n283 = Multiply(x=w447, y=w571) -> (x*y=w557:dbl)
        n284 = Multiply(x=w565, y=w564) -> (x*y=w559:dbl)
        n285 = Unbundle(w452) -> ("Left"=w459:i32, "Top"=w464:i32)
        n286 = Unbundle(w466) -> ("Left"=w473:i32, "Top"=w478:i32)
        n287 = Unbundle(w449) -> ("Left"=w486:i32, "Top"=w491:i32)
        n288 = Unbundle(w493) -> ("Left"=w495:i32, "Top"=w494:i32)
        n289 = Unbundle(w521) -> ("Left"=w528:i32, "Top"=w533:i32)
        n290 = Multiply(x=w557, y=1.0) -> (x*y=w558:dbl)
        n291 = Multiply(x=w559, y=1.0) -> (x*y=w560:dbl)
        n292 = local read "test"() -> (w428:dbl)
        n293 = Subtract(x=w533, y=34) -> (x-y=w529:i32)
        n294 = Add(x=w446, y=w558) -> (x+y=w450:dbl)
        n295 = Add(x=w563, y=w560) -> (x+y=w451:dbl)
        n296 = Add(x=w459, y=38) -> (x+y=w463:i32)
        n297 = Subtract(x=w459, y=34) -> (x-y=w458:i32)
        n298 = Add(x=w464, y=38) -> (x+y=w462:i32)
        n299 = Subtract(x=w464, y=34) -> (x-y=w460:i32)
        n300 = Add(x=w473, y=38) -> (x+y=w477:i32)
        n301 = Subtract(x=w473, y=34) -> (x-y=w472:i32)
        n302 = Add(x=w478, y=38) -> (x+y=w476:i32)
        n303 = Subtract(x=w478, y=34) -> (x-y=w474:i32)
        n304 = Add(x=w486, y=38) -> (x+y=w490:i32)
        n305 = Subtract(x=w486, y=34) -> (x-y=w485:i32)
        n306 = Add(x=w491, y=38) -> (x+y=w489:i32)
        n307 = Subtract(x=w491, y=34) -> (x-y=w487:i32)
        n308 = Add(x=w495, y=38) -> (x+y=w505:i32)
        n309 = Subtract(x=w495, y=34) -> (x-y=w501:i32)
        n310 = Add(x=w494, y=38) -> (x+y=w504:i32)
        n311 = Subtract(x=w494, y=34) -> (x-y=w502:i32)
        n312 = Add(x=w528, y=38) -> (x+y=w532:i32)
        n313 = Subtract(x=w528, y=34) -> (x-y=w527:i32)
        n314 = Add(x=w533, y=38) -> (x+y=w531:i32)
        n315 = In Range and Coerce(upper limit=w463, x=w450, lower limit=w458) -> (In Range?=w454:bool)  [unwired: 1 out]
        n316 = In Range and Coerce(upper limit=w462, x=w451, lower limit=w460) -> (In Range?=w455:bool)  [unwired: 1 out]
        n317 = In Range and Coerce(upper limit=w477, x=w450, lower limit=w472) -> (In Range?=w468:bool)  [unwired: 1 out]
        n318 = In Range and Coerce(upper limit=w476, x=w451, lower limit=w474) -> (In Range?=w469:bool)  [unwired: 1 out]
        n319 = In Range and Coerce(upper limit=w490, x=w450, lower limit=w485) -> (In Range?=w481:bool)  [unwired: 1 out]
        n320 = In Range and Coerce(upper limit=w489, x=w451, lower limit=w487) -> (In Range?=w482:bool)  [unwired: 1 out]
        n321 = In Range and Coerce(upper limit=w505, x=w450, lower limit=w501) -> (In Range?=w497:bool)  [unwired: 1 out]
        n322 = In Range and Coerce(upper limit=w504, x=w451, lower limit=w502) -> (In Range?=w498:bool)  [unwired: 1 out]
        n323 = Bundle(w450, w451) -> (w556:cluster{dbl, dbl})  [unwired: 1 in]
        n324 = In Range and Coerce(upper limit=w532, x=w450, lower limit=w527) -> (In Range?=w523:bool)  [unwired: 1 out]
        n325 = In Range and Coerce(upper limit=w531, x=w451, lower limit=w529) -> (In Range?=w524:bool)  [unwired: 1 out]
        n326 = Equal To 0?(x=w428) -> (x = 0?=w426:bool)
        n327 = property on="Ball" class="Bool (strict)"("Position"=w556) -> ()  [unwired: 2 in, 2 out]
        n328 = And(x=w454, y=w455) -> (x .and. y?=w453:bool)
        n329 = And(x=w468, y=w469) -> (x .and. y?=w467:bool)
        n330 = And(x=w481, y=w482) -> (x .and. y?=w480:bool)
        n331 = And(x=w497, y=w498) -> (x .and. y?=w496:bool)
        n332 = And(x=w523, y=w524) -> (x .and. y?=w516:bool)
        n333 = Select(t=1.0, s=w453, f=0.0) -> (s? t:f=w543:dbl)
        n334 = Select(t=1.0, s=w467, f=0.0) -> (s? t:f=w542:dbl)
        n335 = Select(t=1.0, s=w496, f=0.0) -> (s? t:f=w515:dbl)
        n336 = Select(t=-10.0, s=w480, f=0.0) -> (s? t:f=w541:dbl)
        n337 = Select(t=-10.0, s=w516, f=0.0) -> (s? t:f=w514:dbl)
        n338 = Select(t=T1 {"Left"=50, "Top"=-600}, s=w467, f=w466) -> (s? t:f=w551:T1)
        n339 = Select(t=T1 {"Left"=100, "Top"=-600}, s=w480, f=w449) -> (s? t:f=w550:T1)
        n340 = Select(t=T1 {"Left"=0, "Top"=-600}, s=w453, f=w452) -> (s? t:f=w554:T1)
        n341 = Select(t=T1 {"Left"=200, "Top"=-600}, s=w516, f=w521) -> (s? t:f=w512:T1)
        n342 = Select(t=T1 {"Left"=150, "Top"=-600}, s=w496, f=w493) -> (s? t:f=w513:T1)
        n343 = Compound Arithmetic op=ADD(w540, w543, w542, w541, w515, w514) -> (w429:dbl)
        "judge2" <- w429
        n344 = property on="bowling2" class="Bool (strict)"("Position"=w551) -> ()  [unwired: 2 in, 2 out]
        n345 = property on="bowling3" class="Bool (strict)"("Position"=w550) -> ()  [unwired: 2 in, 2 out]
        n346 = property on="bowling1" class="Bool (strict)"("Position"=w554) -> ()  [unwired: 2 in, 2 out]
        n347 = property on="bowling5" class="Bool (strict)"("Position"=w512) -> ()  [unwired: 2 in, 2 out]
        n348 = property on="bowling4" class="Bool (strict)"("Position"=w513) -> ()  [unwired: 2 in, 2 out]
        n349 = Equal?(x=w432, y=2.0) -> (x = y?=w436:bool)
        n350 = Less Or Equal?(x=w429, y=-16.0) -> (x <= y?=w427:bool)
        n351 = And(x=w427, y=w426) -> (x .and. y?=w425:bool)
        n352 = case shown="True" w425 {
          frame False {
          }
          frame True {
            n353 = One Button Dialog(message="出局啦     \n再試一次吧！     ") -> ()  [unwired: 1 in, 1 out]
          }
        }
        n354 = local read "stop"() -> (w435:bool)
        n355 = Compound Arithmetic op=OR(w436, w427, w435) -> (w437:bool)
      }
    }
    frame #6 {
      n356 = local read "撞擊次數2"() -> (w600:dbl)
      n357 = local read "撞擊次數1"() -> (w601:dbl)
      n358 = local read "judge2"() -> (w581:dbl)
      n359 = local read "選擇的模式1"() -> (w592:dbl)
      n360 = local read "選擇的模式2"() -> (w589:dbl)
      n361 = local read "碰撞次數(以內)"() -> (w599:dbl)
      n362 = local read "時間"() -> (w580:dbl)
      n363 = local read "stop"() -> (w612:bool)
      n364 = Add(x=w601, y=w600) -> (x+y=w598:dbl)
      n365 = Less?(x=w581, y=-16.0) -> (x < y?=w585:bool)
      n366 = Multiply(x=w589, y=30.0) -> (x*y=w587:dbl)
      n367 = Multiply(x=w592, y=50.0) -> (x*y=w590:dbl)
      n368 = Reciprocal(x=w580) -> (1/x=w614:dbl)
      n369 = Select(t=0.0, s=w612, f=1.0) -> (s? t:f=w604:dbl)
      n370 = Subtract(x=w599, y=w598) -> (x-y=w597:dbl)
      n371 = local read "最佳成績"() -> (w613:dbl)
      n372 = case shown="-7" w581 {
        tunnel: [0.0 ("y") 50.0 ("y") 100.0 ("y") 60.0 ("y") 40.0 ("y") 10.0 ("y") -50.0 ("y") 150.0 ("y")] -> w582
        frame 0, Default {
        }
        frame 1 {
        }
        frame 2 {
        }
        frame -7 {
        }
        frame -8 {
        }
        frame -9 {
        }
        frame -10 {
        }
        frame 3 {
        }
      }
      n373 = Select(t=-9999.0, s=w585, f=w582) -> (s? t:f=w583:dbl)
      n374 = Greater Or Equal To 0?(x=w597) -> (x >= 0?=w596:bool)
      n375 = Multiply(x=w614, y=500.0) -> (x*y=w609:dbl)
      n376 = Multiply(x=w590, y=w604) -> (x*y=w605:dbl)
      n377 = Multiply(x=w587, y=w604) -> (x*y=w606:dbl)
      n378 = Multiply(x=w583, y=w604) -> (x*y=w607:dbl)
      n379 = Select(t=50.0, s=w596, f=0.0) -> (s? t:f=w593:dbl)
      n380 = Multiply(x=w609, y=w604) -> (x*y=w608:dbl)
      n381 = Multiply(x=w593, y=w604) -> (x*y=w603:dbl)
      n382 = Compound Arithmetic op=ADD(w603, w605, w606, w607, w608) -> (w602:dbl)
      "分數" <- w602
      n383 = while {
        shift-right: [w625] -> _
        shift-left: w613 -> [w626]
        tunnel: w602 -> [w624]
        stop <- TRUE stop-if-true
        n384 = Greater?(x=w624, y=w626) -> (0:w627:bool)
        n385 = Select(t=w624, s=w627, f=w626) -> (s? t:f=w625:dbl)
        "最佳成績" <- w625
      }
    }
  }
  "bowling1" <- w1
  "bowling2" <- w1
  "bowling3" <- w1
  "Ball" <- w1
  "bowling4" <- w1
  "bowling5" <- w1
